vi "keccak.ip.fifo.control.export.ip.vi"(0 "Reset":bool, 1 "TS_RESULTS.Ready":bool, 2 "TS_PARMS.Element":u64, 3 "TS_PARMS.Valid":bool, 4 "TS_DATA.Element":u64, 5 "TS_DATA.Valid":bool) -> (14 "TS_RESULTS.Element":u64, 15 "TS_RESULTS.Valid":bool, 16 "TS_PARMS.Ready":bool, 17 "TS_DATA.Ready":bool)   [LabVIEW 2021]
uses:
  <vilib>/Platform/TimedLoop/XDataNode/timing_clust.ctl
  <vilib>/Platform/TimedLoop/XDataNode/nitl_modes.ctl
  <vilib>/Platform/TimedLoop/XDataNode/wakeup.ctl
  <vilib>/rvi/Emulation/niFpgaSctlEmulationGetInTimedLoop.vi
  <vilib>/rvi/Emulation/niFpgaEmulationReportErrorSimple.vi
  <vilib>/rvi/Emulation/niFpgaGetClockAttributes.vi
  <vilib>/rvi/Emulation/niFpgaCriticalErrorInLSC.vi
  <vilib>/platform/TimedLoop/XDataNode/XDataNode.xnode
  <vilib>/Platform/TimedLoop/XDataNode/XDNodeRunTimeDep.lvlib
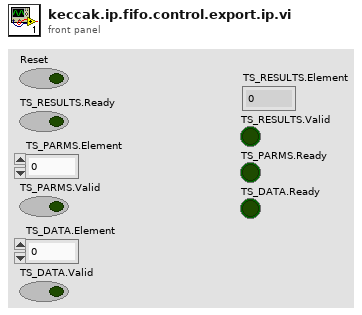
[diagram p1: front panel]
types:
  T1 = typedef "XDNodeRunTimeDep.lvlib/timing_clust.ctl" = cluster{"Expected End [f-1]":u64, "Actual End [f-1]":u64, "Finished Late? [f-1]":bool, "Expected End [i-1]":u64, "Actual End [i-1]":u64, "Finished Late? [i-1]":bool, "Expected Start [i]":u64, "Actual Start [i]":u64, "Expected Start [f]":u64, "Actual Start [f]":u64, "Source Name":string, "Structure Name":string, "Period":i64, "Deadline":i64, "Offset":i64, "Start":i64, "Priority":i32, "Timeout":i32, "Mode":T2, "Wakeup Reason":T3, "Error":errorcluster, "Source Type":string, "Secondary Source Type":string, "Global End Time":u64, "Global Start Time":u64, "Frame Duration":u64, "Iteration Duration":u64, "Assigned CPU":i32, "I/O Scan Engine Mode":u32}
  T2 = typedef "XDNodeRunTimeDep.lvlib/nitl_modes.ctl" = enum32{"No Change", "Process missed periods, maintain original phase", "Discard missed periods, maintain original phase", "Process missed periods, ignore original phase", "Discard missed periods, ignore original phase"}
  T3 = typedef "XDNodeRunTimeDep.lvlib/wakeup.ctl" = enum32{"Normal", "Aborted", "Asynchronous wakeup", "Timing source error", "Timed loop error", "Timeout"}
  T4 = cluster{"TS_RESULTS.Ready":bool, "TS_PARMS.Element":u64, "TS_PARMS.Valid":bool, "TS_DATA.Element":u64, "TS_DATA.Valid":bool}
  T5 = cluster{"TS_RESULTS.Element":u64, "TS_RESULTS.Valid":bool, "TS_PARMS.Ready":bool, "TS_DATA.Ready":bool}
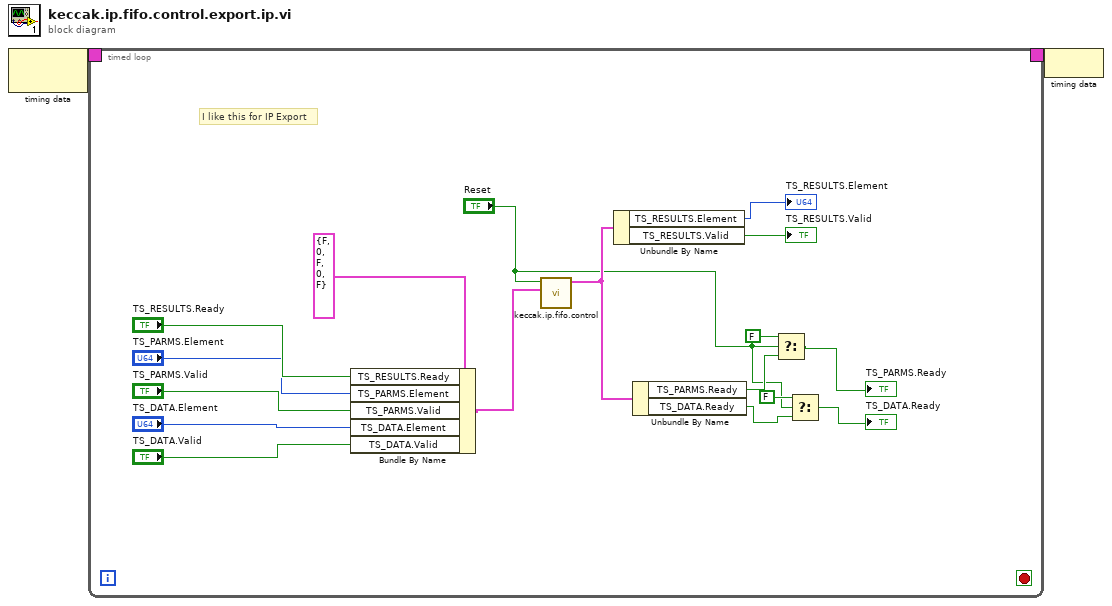
[diagram p0: block diagram]
diagram:
  n1 = node-c288() -> (w2:T1)  [unwired: 1 in]
  n2 = timed-loop {
    timing: w2 -> [_]
    timing-out: [_] -> w1
    stop <- _ stop-if-true
    # "I like this for IP Export"
    n3 = Bundle By Name(cluster=T4 {"TS_RESULTS.Ready"=FALSE, "TS_PARMS.Element"=0, "TS_PARMS.Valid"=FALSE, "TS_DATA.Element"=0, "TS_DATA.Valid"=FALSE} ("FIFO.inputs"), "TS_RESULTS.Ready"="TS_RESULTS.Ready", "TS_PARMS.Element"="TS_PARMS.Element", "TS_PARMS.Valid"="TS_PARMS.Valid", "TS_DATA.Element"="TS_DATA.Element", "TS_DATA.Valid"="TS_DATA.Valid") -> (w15:T4)
    n4 = call "keccak.ip.fifo.control.vi"("FIFO.inputs"=w15, "Reset"="Reset") -> ("FIFO.outputs"=w19:T5)  [unwired: 9 in]
    n5 = Unbundle By Name(w19) -> ("TS_RESULTS.Element"=→"TS_RESULTS.Element":u64, "TS_RESULTS.Valid"=→"TS_RESULTS.Valid":bool)
    n6 = Unbundle By Name(w19) -> ("TS_PARMS.Ready"=w9:bool, "TS_DATA.Ready"=w6:bool)
    n7 = Select(t=FALSE, s="Reset", f=w9) -> (s? t:f=→"TS_PARMS.Ready":bool)
    n8 = Select(t=FALSE, s="Reset", f=w6) -> (s? t:f=→"TS_DATA.Ready":bool)
  }
  n9 = node-c288(w1) -> ()
